vi "CallConfig.vi"(5 "Number of Bytes to Read":u8, 6 "Time out?":u8=10, 7 "Number of Bytes to Write":u8, 8 "error in (no error)":errorcluster, 10 "Command":enum16{"Write", "Read", "Write&Read"}(ring), 11 "FPGA VI引用输入":refnum<k20>) -> (0 "error out":errorcluster, 3 "FPGA VI引用输出":refnum<k20>)   [LabVIEW 2015]
uses:
  <vilib>/Utility/error.llb/Error Cluster From Error Code.vi
  <vilib>/rvi/errors/niLvFpgaAdjustHostInterfaceError.vi
  <vilib>/rvi/interface/nirviReadWriteControl/nirviReadWriteControl.xnode
  <vilib>/rvi/interface/Simulation/niFpgaSimulationCallBeginRW.vi
  NiFpgaLv.dll
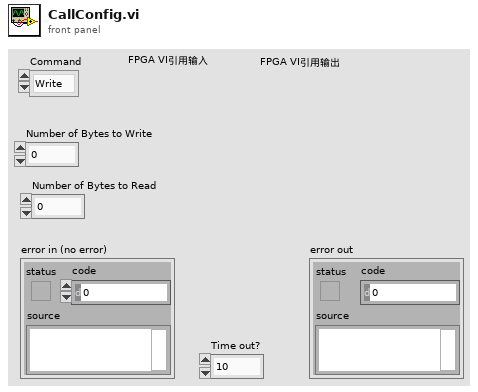
[diagram p1: front panel]
types:
  T1 = enum8{"IDLE", "SetIDLE", "Config", "Arm", "Read", "Write", "AutoRead"}
  T2 = cluster{"WriteNumber":u8, "ReadNumber":u8, "CMD":enum8{"Write & Read", "Write", "Read"}}
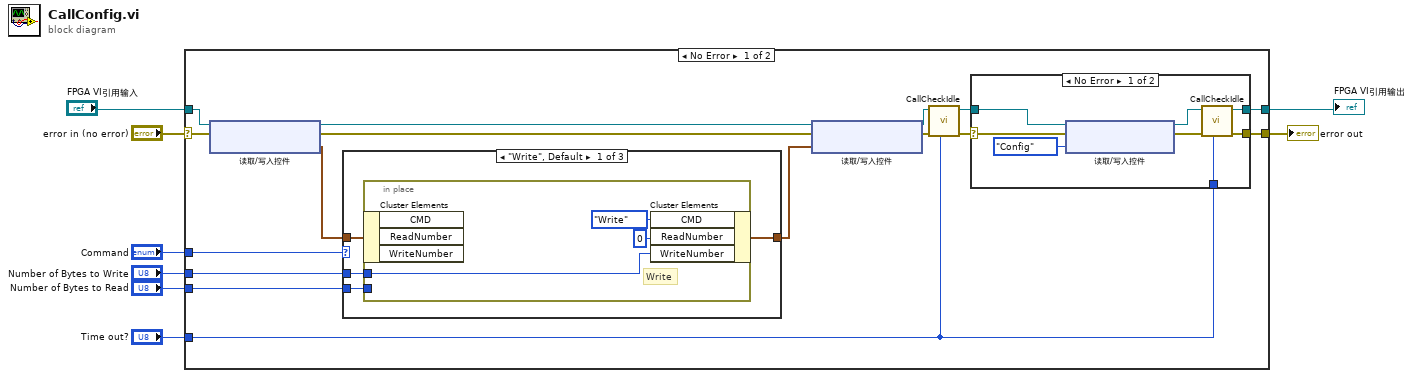
[diagram p0: block diagram]
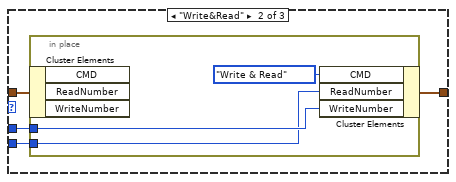
[diagram p3: hidden frame]
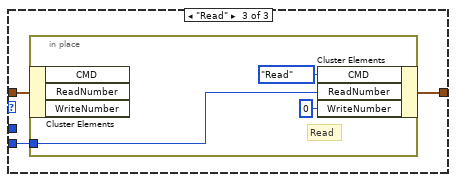
[diagram p4: hidden frame]
diagram:
  n1 = case shown="No Error" "error in (no error)" {
    selector: "error in (no error)" -> [w22 w56]
    tunnel: "Number of Bytes to Read" -> [w24 _]
    tunnel: [w21 w56] -> w7
    tunnel: "Command" -> [w23 _]
    tunnel: "Time out?" -> [w13 _]
    tunnel: "FPGA VI引用输入" -> [w17 w55]
    tunnel: "Number of Bytes to Write" -> [w10 _]
    tunnel: [w9 w55] -> w1
    frame No Error {
      n2 = xnode "读取/写入控件"("FPGA VI Reference In"=w17, "error in"=w22) -> ("FPGA VI Reference Out"=w19:refnum<k20>, "error out"=w20:errorcluster, "CMDParameters"=w18:T2)
      n3 = case shown="\"Write\", Default" w23 {
        tunnel: w24 -> [w38 w45 w51]
        tunnel: [w37 w44 w50] -> w16
        tunnel: w18 -> [w36 w43 w49]
        tunnel: w10 -> [w35 w42 _]
        frame "Write", Default {
          n4 = in-place {
            in-place-border: w38 -> [_]
            in-place-border: w35 -> [w39]
            # "Write"
            n5 = in-place-cluster #1(w36) -> ()  [unwired: 3 out]
            n6 = in-place-cluster #1("CMD"=enum8{"Write & Read", "Write", "Read"}."Write", "ReadNumber"=u8 0, "WriteNumber"=w39) -> (w37:T2)
          }
        }
        frame "Write&Read" {
          n7 = in-place {
            in-place-border: w45 -> [w46]
            in-place-border: w42 -> [w47]
            n8 = in-place-cluster #2(w43) -> ()  [unwired: 3 out]
            n9 = in-place-cluster #2("CMD"=enum8{"Write & Read", "Write", "Read"}."Write & Read", "ReadNumber"=w46, "WriteNumber"=w47) -> (w44:T2)
          }
        }
        frame "Read" {
          n10 = in-place {
            in-place-border: w51 -> [w54]
            # "Read"
            n11 = in-place-cluster #3(w49) -> ()  [unwired: 3 out]
            n12 = in-place-cluster #3("CMD"=enum8{"Write & Read", "Write", "Read"}."Read", "ReadNumber"=w54, "WriteNumber"=u8 0) -> (w50:T2)
          }
        }
      }
      n13 = xnode "读取/写入控件"("FPGA VI Reference In"=w19, "error in"=w20, "CMDParameters"=w16) -> ("FPGA VI Reference Out"=w12:refnum<k20>, "error out"=w15:errorcluster)
      n14 = call "CallCheckIdle.vi"("Time out?"=w13, "error in (no error)"=w15, "FPGA VI引用输入"=w12) -> ("error out"=w14:errorcluster, "FPGA VI引用输出"=w11:refnum<k20>)  [unwired: 7 in]
      n15 = case shown="No Error" w14 {
        selector: w14 -> [w31 w34]
        tunnel: w11 -> [w32 w33]
        tunnel: [w29 w34] -> w21
        tunnel: w13 -> [w27 _]
        tunnel: [w25 w33] -> w9
        frame No Error {
          n16 = xnode "读取/写入控件"("FPGA VI Reference In"=w32, "error in"=w31, "ProtocolControl"=T1."Config") -> ("FPGA VI Reference Out"=w26:refnum<k20>, "error out"=w28:errorcluster)
          n17 = call "CallCheckIdle.vi"("Time out?"=w27, "error in (no error)"=w28, "FPGA VI引用输入"=w26) -> ("error out"=w29:errorcluster, "FPGA VI引用输出"=w25:refnum<k20>)  [unwired: 7 in]
        }
        frame Error {
        }
      }
    }
    frame Error {
    }
  }
  "error out" <- w7
  "FPGA VI引用输出" <- w1
